vi "self-resetting-iter-TEST.vi"() -> (1 "Numeric":i32)   [LabVIEW 2015]
uses:
  <vilib>/rvi/Emulation/niFpgaGetClockAttributes.vi
  <vilib>/rvi/Emulation/niFpgaSctlEmulationGetInTimedLoop.vi
  <vilib>/rvi/Emulation/niFpgaEmulationReportErrorSimple.vi
  <vilib>/rvi/Emulation/niFpgaCriticalErrorInLSC.vi
  libimaging-cs.lvlib
panel:
  in  "outer-iter-max":i32=2
  out "Array 2":i16[](array[numeric])
  out "Array":bool[](array[boolean])
  in  "zup-N":i16
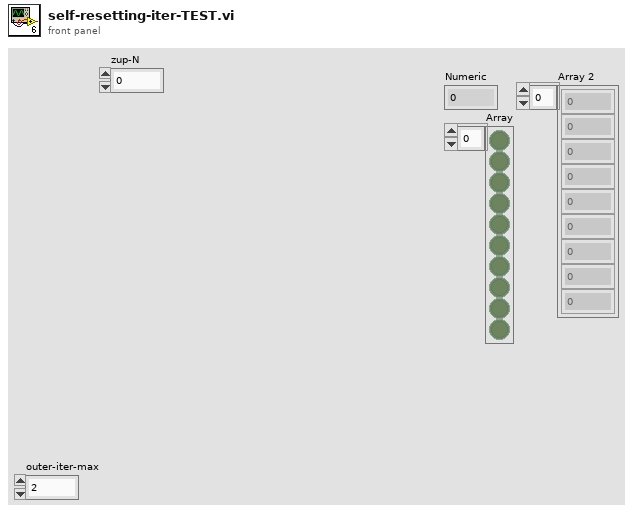
[diagram p1: front panel]
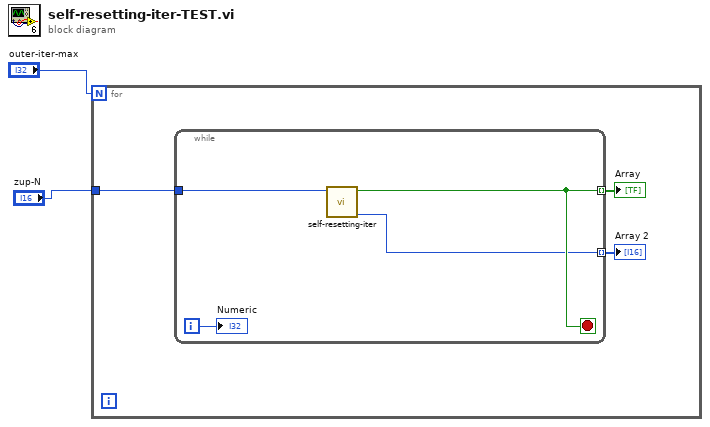
[diagram p0: block diagram]
diagram:
  n1 = for {
    N: "outer-iter-max" -> [_]
    tunnel: "zup-N" -> [w3]
    n2 = while {
      tunnel: [w8] -> w5 mode=indexing
      tunnel: [w7] -> w4 mode=indexing
      tunnel: w3 -> [w6]
      i -> [w9]
      stop <- w8 stop-if-true
      n3 = call "self-resetting-iter.vi"("zup-N"=w6) -> ("Numeric"=w7:i16, "Boolean"=w8:bool)  [unwired: 9 in]
      "Numeric" <- w9
    }
    "Array" <- w5
    "Array 2" <- w4
  }
